vi "SSL Detection Ball Closest.vi"(10 "Ball Array":T1[](array[typedef]), 11 "Detection Ball":T1) -> (0 "Closest index(es)":i32, 1 "Dist":dbl, 2 "Ball Array Out":T1[](array[typedef]), 3 "element":T1)   [LabVIEW 2016]
uses:
  SSL Detection Ball.ctl
  <vilib>/Analysis/_algsub.llb/Vector Norm Type.ctl
  <vilib>/Analysis/_algsub.llb/Real Vector Norm.vi
  <vilib>/Analysis/NI_AALPro.lvlib
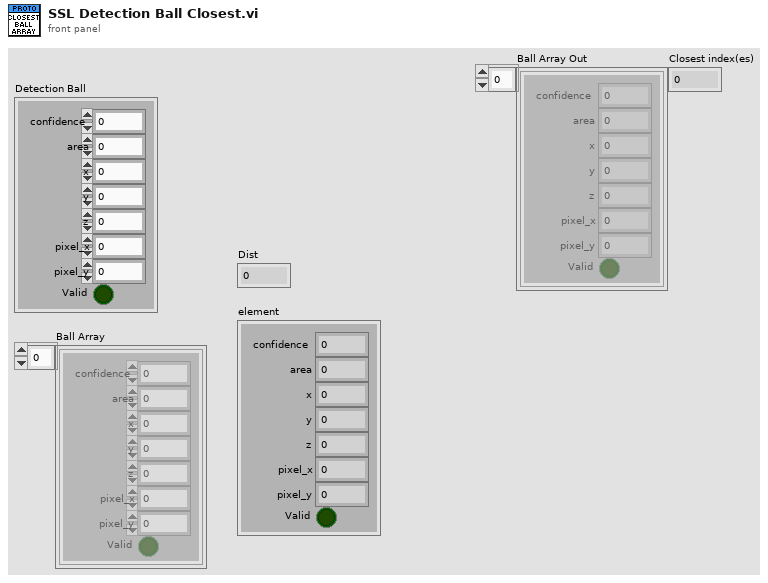
[diagram p1: front panel]
types:
  T1 = typedef "SSL Detection Ball.ctl" = cluster{"x":sgl, "area":u32, "confidence":sgl, "y":sgl, "z":sgl, "pixel_x":sgl, "pixel_y":sgl, "Valid":bool}
  T2 = typedef "NI_AALPro.lvlib/Vector Norm Type.ctl" = u16
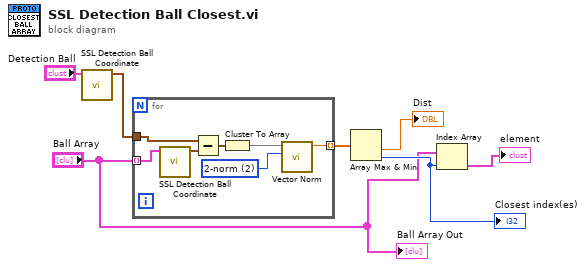
[diagram p0: block diagram]
diagram:
  n1 = call "SSL Detection Ball Coordinate.vi"("Detection Ball"="Detection Ball") -> ("Coordinate"=w2:cluster{"x":sgl, "y":sgl, "z":sgl})  [unwired: 10 in]
  n2 = for {
    tunnel: "Ball Array" -> [w14] mode=indexing
    tunnel: w2 -> [w12]
    tunnel: [w8] -> w3 mode=indexing
    w9 = T2 2 items=["1-norm"=1, "2-norm"=2, "Inf-norm"=3, "-Inf-norm"=4, "User Defined"=5] ("norm type")
    n3 = call "SSL Detection Ball Coordinate.vi"("Detection Ball"=w14) -> ("Coordinate"=w13:cluster{"x":sgl, "y":sgl, "z":sgl})  [unwired: 10 in]
    n4 = Subtract(x=w12, y=w13) -> (x-y=w11:cluster{"x":sgl, "y":sgl, "z":sgl})
    n5 = Cluster To Array(cluster=w11) -> (array=w10:sgl[])
    n6 = call-poly <vilib>:"Vector Norm.vi"("norm type"=w9, "Input Vector"=w10) -> ("norm"=w8:dbl)  [unwired: 8 in, 1 out]
  }
  n7 = Array Max & Min(array=w3) -> (min value=→"Dist":dbl, min index (indices)=w5:i32)  [unwired: 2 out]
  "Closest index(es)" <- w5
  n8 = Index Array(array="Ball Array", index=w5) -> (element=→"element":T1)
  "Ball Array Out" <- "Ball Array"
